vi "Lezeti_Power_Monitor_22_d.vi"() -> ()   [LabVIEW 2014]
uses:
  <vilib>/measure/madcrms.llb/Basic Averaged DC-RMS for N Chan.vi
  <vilib>/measure/madcrms.llb/Basic Averaged DC-RMS for 1 Chan.vi
  <vilib>/Utility/file.llb/Write To Spreadsheet File (DBL).vi
  <vilib>/measure/NI_MAPro.lvlib
panel:
  in  "High Resolution Waveform Data Path":path
  out "Power Factor":dbl
  in  "Average Power Output File":path
  out "Run Date":string
  out "Run Time":string
  out "Elapsed Time (s)":dbl
  out "Apparent Power (VA)":dbl
  out "Average Power (Watts)":dbl
  out "Instantaneous Power Waveform":waveform(dbl)[](graph)
  out "RMS Voltage L1-L2":dbl
  out "L2 RMS Current":dbl
  out "L1 RMS Current":dbl
  in  "Burden Resistor (ohms) (1000)":dbl
  in  "CT Ratio (Iout/Iin) (.0003332)":dbl
  in  "Acquire Sample Size (1000)":dbl
  in  "Acquire Rate (Hz) (1000)":dbl
  in  "Acquire Timeout (1000)":dbl
  out "Line 2 Current Waveform":waveform(dbl)[](graph)
  out "Line 1 Current Waveform":waveform(dbl)[](graph)
  out "Voltage L1-L2":waveform(dbl)[](graph)
  in  "stop":bool
  # "For Lezeti Air Conditioning System (Greenpath Tech)\nBy Matsu Thornton\nJuly 2016"
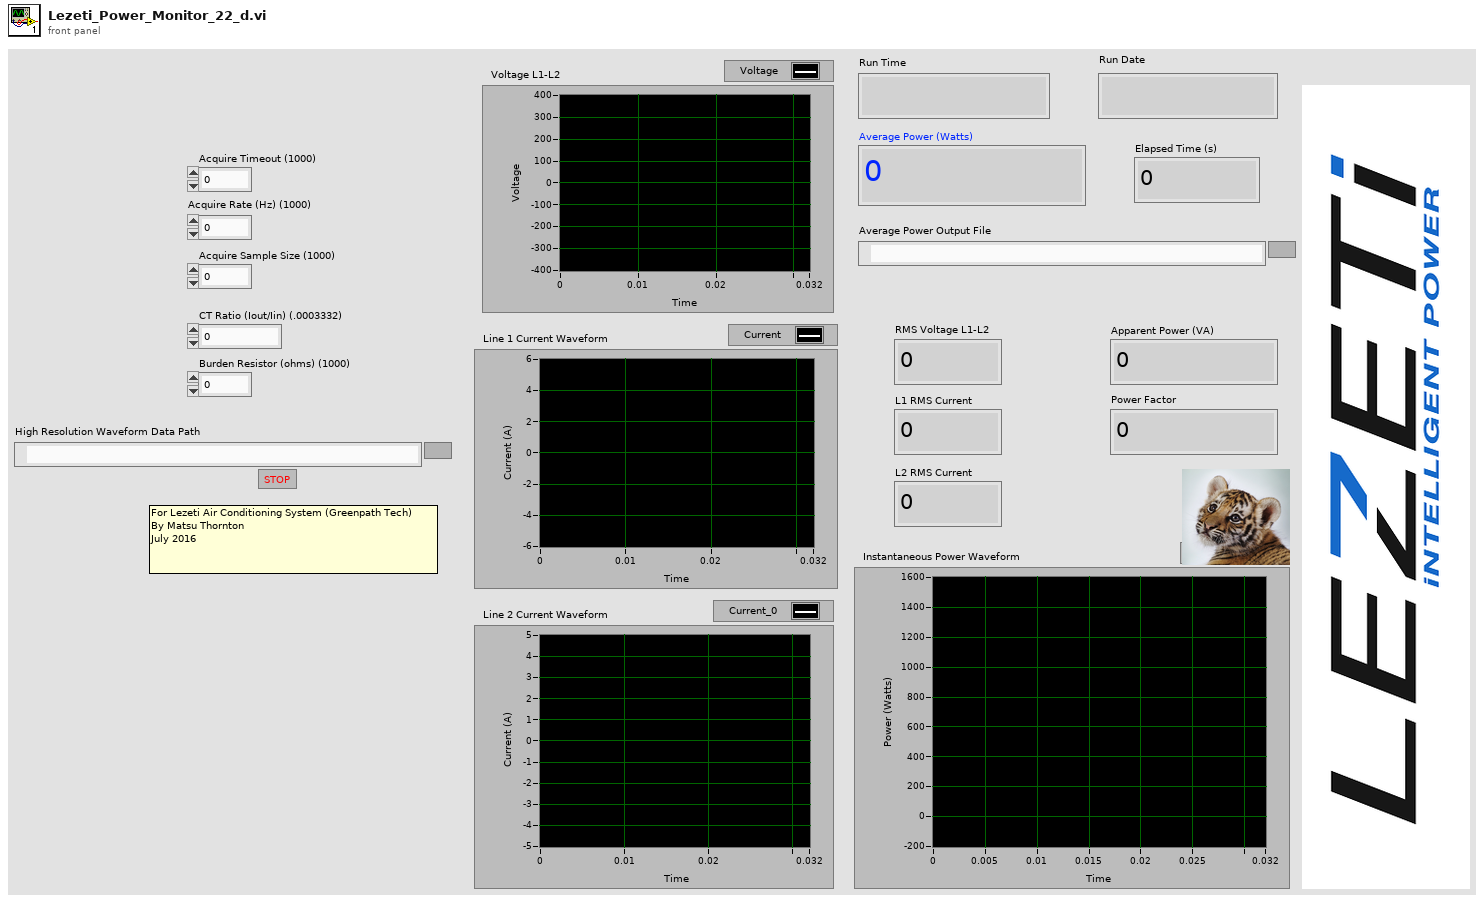
[diagram p1: front panel]
types:
  T1 = typedef "NI_Matrix.lvlib/RealMatrix.ctl" = dbl[][]
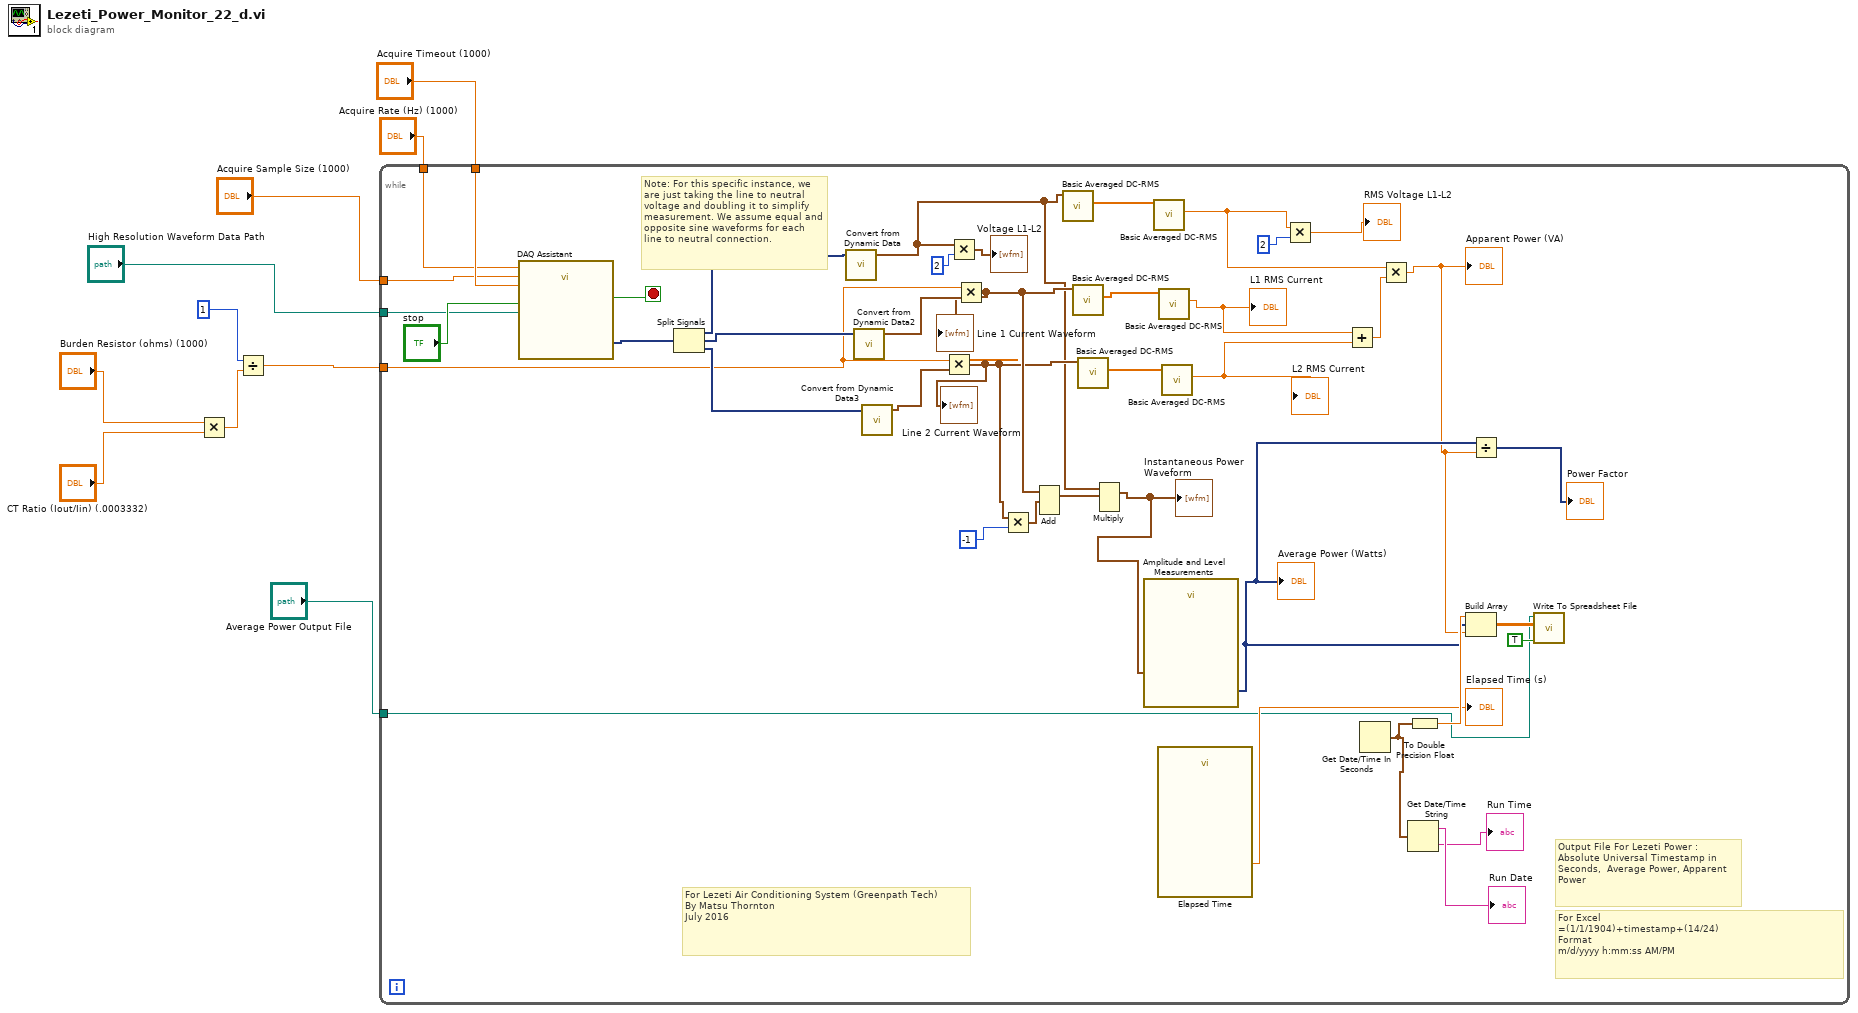
[diagram p0: block diagram]
diagram:
  n1 = Multiply(x="Burden Resistor (ohms) (1000)", y="CT Ratio (Iout/Iin) (.0003332)") -> (x*y=w4:dbl)
  n2 = Divide(x=1, y=w4) -> (x/y=w3:dbl)
  n3 = while {
    tunnel: "Acquire Timeout (1000)" -> [w48]
    tunnel: "Acquire Rate (Hz) (1000)" -> [w24]
    tunnel: "Acquire Sample Size (1000)" -> [w23]
    tunnel: w3 -> [w43]
    tunnel: "Average Power Output File" -> [w27]
    tunnel: "High Resolution Waveform Data Path" -> [w22]
    stop <- w21 stop-if-true
    # "Note: For this specific instance, we are just taking the line to neutral voltage and doubling it to simplify measurement. We assume equal and opposite sine waveforms for each line to neutral connection."
    # "For Excel\n=(1/1/1904)+timestamp+(14/24)\nFormat\nm/d/yyyy h:mm:ss AM/PM"
    # "Output File For Lezeti Power :\nAbsolute Universal Timestamp in Seconds,  Average Power, Apparent Power"
    # "For Lezeti Air Conditioning System (Greenpath Tech)\nBy Matsu Thornton\nJuly 2016"
    n4 = call "DAQ Assistant"("rate"=w24, "number of samples"=w23, "timeout (s)"=w48, "stop (F)"="stop", "file path"=w22) -> ("data"=w52:dynamicdata, "stopped"=w21:bool)  [unwired: 11 in, 2 out]
    n5 = Split Signals(w52) -> (w51:dynamicdata, w50:dynamicdata, w49:dynamicdata)  [unwired: 3 in]
    n6 = call "Convert from Dynamic Data"("Dynamic Data Type"=w51) -> ("Array of Waveform"=w12:waveform(dbl)[])  [unwired: 3 in]
    n7 = call "Convert from Dynamic Data2"("Dynamic Data Type"=w50) -> ("Array of Waveform"=w42:waveform(dbl)[])  [unwired: 3 in]
    n8 = call "Convert from Dynamic Data3"("Dynamic Data Type"=w49) -> ("Array of Waveform"=w41:waveform(dbl)[])  [unwired: 3 in]
    n9 = Multiply(x=w43, y=w41) -> (x*y=w19:waveform(dbl)[])
    "Line 2 Current Waveform" <- w19
    n10 = Multiply(x=w12, y=2) -> (x*y=→"Voltage L1-L2":waveform(dbl)[])
    n11 = Multiply(x=w43, y=w42) -> (x*y=w38:waveform(dbl)[])
    "Line 1 Current Waveform" <- w38
    n12 = Multiply(x=w19, y=-1) -> (x*y=w20:waveform(dbl)[])
    n13 = Add(1:w20, 2:w38) -> (0:w40:waveform(dbl)[])  [unwired: 1 in, 1 out]
    n14 = call-poly <vilib>:"Basic Averaged DC-RMS.vi"("signals in"=w12) -> ("RMS values"=w46:dbl[])  [unwired: 7 in, 3 out]
    n15 = call-poly <vilib>:"Basic Averaged DC-RMS.vi"("signals in"=w38) -> ("RMS values"=w45:dbl[])  [unwired: 7 in, 3 out]
    n16 = call-poly <vilib>:"Basic Averaged DC-RMS.vi"("signals in"=w19) -> ("RMS values"=w44:dbl[])  [unwired: 7 in, 3 out]
    n17 = Multiply(1:w40, 2:w12) -> (0:w39:waveform(dbl)[])  [unwired: 1 in, 1 out]
    "Instantaneous Power Waveform" <- w39
    n18 = call "Amplitude and Level Measurements"("Signals"=w39) -> ("Mean (DC)"=w26:dynamicdata)  [unwired: 13 in, 1 out]
    "Average Power (Watts)" <- w26
    n19 = call-poly <vilib>:"Basic Averaged DC-RMS.vi"("signal in"=w46) -> ("RMS value"=w15:dbl)  [unwired: 7 in, 3 out]
    n20 = call "Elapsed Time"() -> ("Elapsed Time (s)"=→"Elapsed Time (s)":dbl)  [unwired: 12 in, 7 out]
    n21 = call-poly <vilib>:"Basic Averaged DC-RMS.vi"("signal in"=w45) -> ("RMS value"=w37:dbl)  [unwired: 7 in, 3 out]
    "L1 RMS Current" <- w37
    n22 = call-poly <vilib>:"Basic Averaged DC-RMS.vi"("signal in"=w44) -> ("RMS value"=w36:dbl)  [unwired: 7 in, 3 out]
    "L2 RMS Current" <- w36
    n23 = Multiply(x=w15, y=2) -> (x*y=→"RMS Voltage L1-L2":dbl)
    n24 = Add(x=w37, y=w36) -> (x+y=w35:dbl)
    n25 = Get Date/Time In Seconds() -> (seconds since 1Jan1904=w31:timestamp)
    n26 = Multiply(x=w15, y=w35) -> (x*y=w17:dbl)
    "Apparent Power (VA)" <- w17
    n27 = Get Date/Time String(seconds (now)=w31) -> (date string=→"Run Date":string, time string=→"Run Time":string)  [unwired: 2 in]
    n28 = To Double Precision Float(number=w31) -> (double precision float=w32:dbl)
    n29 = Build Array(w32, w26, w17) -> (w33:T1)
    n30 = Divide(x=w26, y=w17) -> (x/y=→"Power Factor":dynamicdata)
    n31 = call-poly <vilib>:"Write To Spreadsheet File.vi"("append to file? (new file:F)"=TRUE, "2D data"=w33, "file path (dialog if empty)"=w27) -> ()  [unwired: 5 in, 1 out]
  }
